vi "TEst FITS Headers.vi"() -> ()   [LabVIEW 2021]
uses:
  <userlib>/gfitsio/gfitsio-read-key-integer.vi
  <userlib>/gfitsio/gfitsio.lvlib
panel:
  out "Array":T1(array[cluster])
  in  "Fields":string[](array[string])
  in  "Folder":path
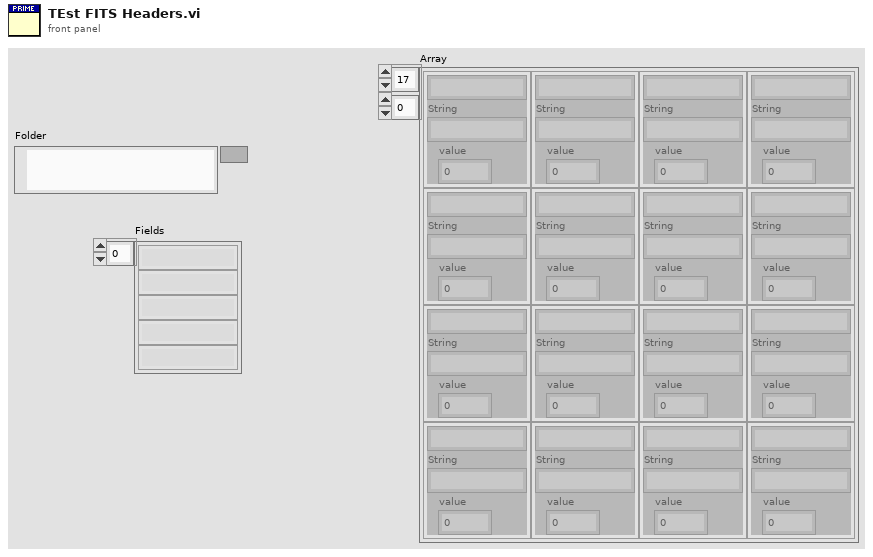
[diagram p1: front panel]
types:
  T1 = cluster{string, "String":string, "value":i32}[][]
  T2 = enum16{"open", "open or create", "create or replace", "create", "open (read only)"}
  T3 = typedef "gfitsio.lvlib/gfitsio-refnum.ctl" = refnum<k1>
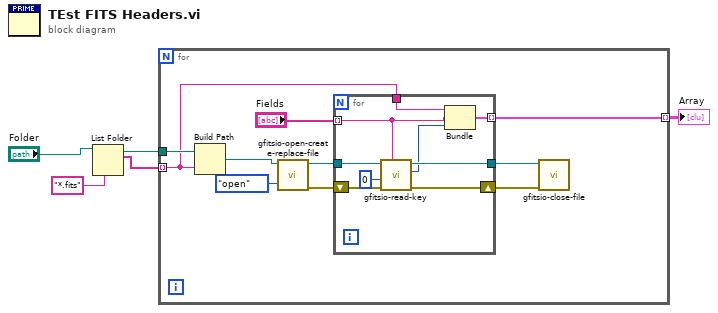
[diagram p0: block diagram]
diagram:
  n1 = List Folder(path="Folder", pattern="*.fits") -> (path out=w3:path, filenames=w2:string[])  [unwired: 2 in, 2 out]
  n2 = for {
    tunnel: w3 -> [w15]
    tunnel: w2 -> [w7] mode=indexing
    tunnel: [w6] -> w1 mode=indexing
    n3 = Build Path(base path=w15, name or relative path=w7) -> (appended path=w14:path)
    n4 = call <userlib>:"gfitsio-open-create-replace-file.vi"("function (open)"=T2."open", "file path (dialog if empty)"=w14) -> ("error out"=w11:errorcluster, "gfits refnum"=w12:T3)  [unwired: 7 in, 1 out]
    n5 = for {
      tunnel: w12 -> [w24]
      shift-right: [w22] -> w9
      shift-left: w11 -> [w23]
      tunnel: "Fields" -> [w18] mode=indexing
      tunnel: [w21] -> w8
      tunnel: w7 -> [w17]
      tunnel: [w16] -> w6 mode=indexing
      n6 = call-poly <userlib>:"gfitsio-read-key.vi"("keyname"=w18, "error in (no error)"=w23, "default value"=0, "gfits refnum"=w24) -> ("error out"=w22:errorcluster, "value"=w19:i32, "dup gfits refnum"=w21:T3)  [unwired: 3 in, 2 out]
      n7 = Bundle(w17, "String"=w18, "value"=w19) -> (w16:cluster{string, "String":string, "value":i32})  [unwired: 1 in]
    }
    n8 = call <userlib>:"gfitsio-close-file.vi"("error in (no error)"=w9, "gfits refnum"=w8) -> ()  [unwired: 8 in, 2 out]
  }
  "Array" <- w1
